vi "Select Known Hosts File.vi"(6 "Default Name":string="known_hosts", 8 "Error In":errorcluster caption="error in", 11 "Start Folder":path=path "") -> (0 "Error Out":errorcluster caption="error out", 3 "Known Hosts File":path)   [LabVIEW 2018, in "Tests.lvlib"]
uses:
  Tests.lvlib
  <vilib>/Utility/sysdir.llb/System Directory Type.ctl
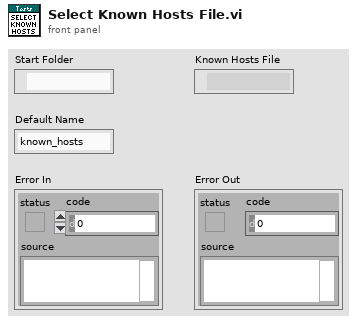
[diagram p1: front panel]
types:
  T1 = typedef "System Directory Type.ctl" = i32
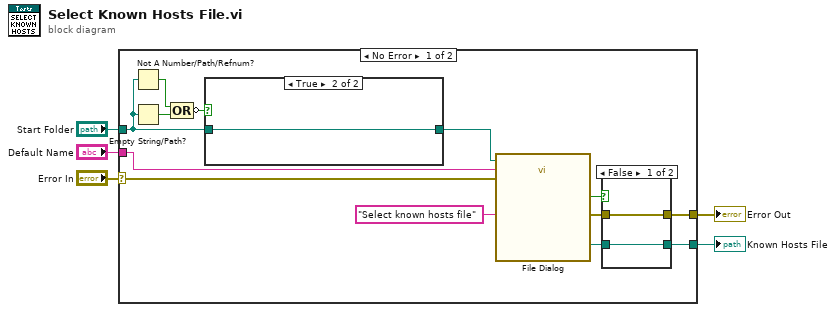
[diagram p0: block diagram]
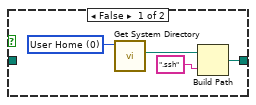
[diagram p2: hidden frame]
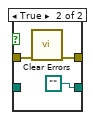
[diagram p3: hidden frame]
diagram:
  n1 = case shown="No Error" "Error In" {
    selector: "Error In" -> [w11 w29]
    tunnel: [w14 w29] -> w5
    tunnel: [w12 _] -> w4
    tunnel: "Default Name" -> [w10 _]
    tunnel: "Start Folder" -> [w7 _]
    frame No Error {
      n2 = Not A Number/Path/Refnum?(number/path/refnum=w7) -> (NaN/Path/Refnum?=w8:bool)
      n3 = Empty String/Path?(string/path=w7) -> (empty?=w9:bool)
      n4 = Compound Arithmetic op=OR(w8, w9) -> (invert w6:bool)
      n5 = case shown="True" w6 {
        tunnel: [w19 w23] -> w18
        tunnel: w7 -> [_ w23]
        frame False {
          w22 = T1 0 items=["User Home"=0, "User Desktop"=1, "User Documents"=2, "User Application Data"=3, "User Preferences"=4, "User Temporary"=5, "Public Documents"=6, "Public Application Data"=7, "Public Preferences"=8, "Public Cache"=13, "System Core Libraries"=9, "System Installed Libraries"=10, "Application Files"=11, "Boot Volume Root"=12] ("system directory type")
          n6 = call <vilib>:"Get System Directory.vi"("system directory type"=w22) -> ("system directory"=w21:path)  [unwired: 10 in]
          n7 = Build Path(base path=w21, name or relative path=".ssh") -> (appended path=w19:path)
        }
        frame True {
        }
      }
      n8 = call "File Dialog"("start path"=w18, "prompt"="Select known hosts file", "default name"=w10, "error in"=w11) -> ("selected path"=w13:path, "cancelled"=w16:bool, "error out"=w15:errorcluster)  [unwired: 8 in, 1 out]
      n9 = case shown="False" w16 {
        tunnel: w15 -> [w25 w28]
        tunnel: [w25 w27] -> w14
        tunnel: w13 -> [w24 _]
        tunnel: [w24 path ""] -> w12
        frame False {
        }
        frame True {
          n10 = call <vilib>:"Clear Errors.vi"("error in (no error)"=w28) -> ("error out"=w27:errorcluster)  [unwired: 5 in, 1 out]
        }
      }
    }
    frame Error {
    }
  }
  "Error Out" <- w5
  "Known Hosts File" <- w4
